vi "Send.vi"(1 "Array":string[][](array[string]), 2 "Topic":string, 3 "MQTT_API in":refnum<class "MQTT_API.lvclass">) -> (0 "MQTT_API out":refnum<class "MQTT_API.lvclass">)   [LabVIEW 2019]
uses:
  <vilib>/addons/WireFlow/_WireQueue/MQTT API/MQTT_API.lvclass
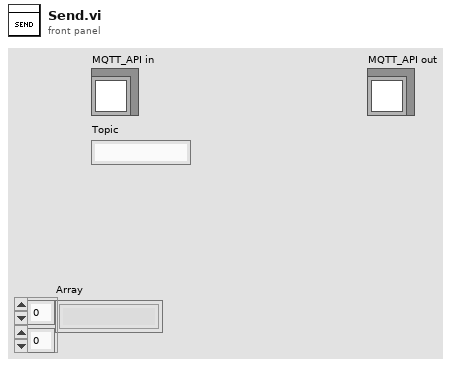
[diagram p1: front panel]
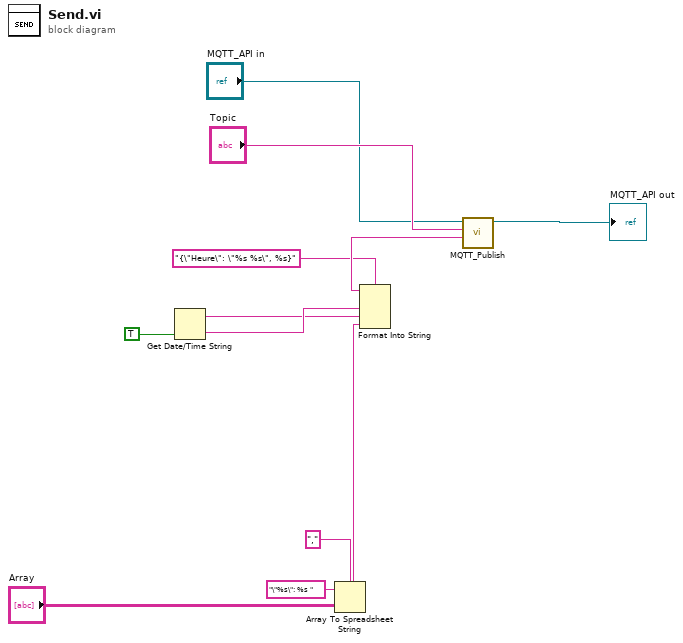
[diagram p0: block diagram]
diagram:
  n1 = Get Date/Time String(want seconds? (F)=TRUE) -> (date string=w6:string, time string=w7:string)  [unwired: 2 in]
  n2 = Array To Spreadsheet String(delimiter (Tab)=",", array="Array", 3:"\"%s\": %s " ("format string")) -> (spreadsheet string=w4:string)
  n3 = Format Into String(format string="{\"Heure\": \"%s %s\", %s}", w7, w6, w4) -> (resulting string=w9:string)  [unwired: 2 in, 1 out]
  n4 = call <vilib>:"MQTT_Publish.vi"("Value"=w9, "Topic name"="Topic", "MQTT_API in"="MQTT_API in") -> ("MQTT_API out"=→"MQTT_API out":refnum<class "MQTT_API.lvclass">)  [unwired: 7 in, 1 out]
